vi "DisplayConfig.vi"(9 "EnableSounds":bool) -> (4 "ScoreIP":string, 6 "Cancelled?":bool, 8 "TimerIP":string, 10 "EnableSounds out":bool, 15 "Score Behavior OUT":T1(ring))   [LabVIEW 2013]
uses:
  <vilib>/httpClient/LabVIEWHTTPClient.lvlib
panel:
  in  "Tab Control":enum32{"Page 1", "Page 2"}(tab)
  in  "Tab Control 2":enum32{"Basic Settings", "Advanced"}(tab)
  in  "IP Address (ex:  127.0.0.1)":string="127.0.0.1"
  in  "Check IP Button":bool
  in  "Port (ex:  8008)":string="8008"
  in  "Configure Sound Button":bool
  in  "Score Behavior":T1(ring)
  in  "Timer IP Addr":string="127.0.0.1"
  in  "MultiHomed Timer":bool
  in  "Process Stop Button":bool
  in  "OK Button":bool
  out "Instructions":string="This is the Display Application configuration utility for the FIRST LEGO League Tournament Software.  \n\nPlease type in the IP Address of the server system in the IP Address box to the left and press the \"Check\" button to verify that the server is running.  \"127.0.0.1\" is the default address for launching this application on the SERVER machine itself.  On the SERVER machine, the IP address can be found in the \"Monitor\" page at the bottom left.\n\nOnce you close this page, you can open this back up by pressing the ESC key.  You can press the SPACEBAR to make the display application expand the page, but the page MUST be on a display that is exactly 1024x768.\n\nThe display, by default, will show negative scores as ZERO while maintaining the negative value (for ranking purposes) within the software.  To show negatives scores at their true value, change the Score Behavior to reflect this.  \n\nThe display can play sounds similar to the server application.  This is a major hack, please only use this if you're using the standard sounds and don't need to change settings (unless you REALLY feel like you know what you're doing).  Currently sounds are only configured if enabled on initial launch of the display.  Sounds and config are NOT currently shared between the server and display, but the config information may be shared if hosted on the same computer.  Use with caution."
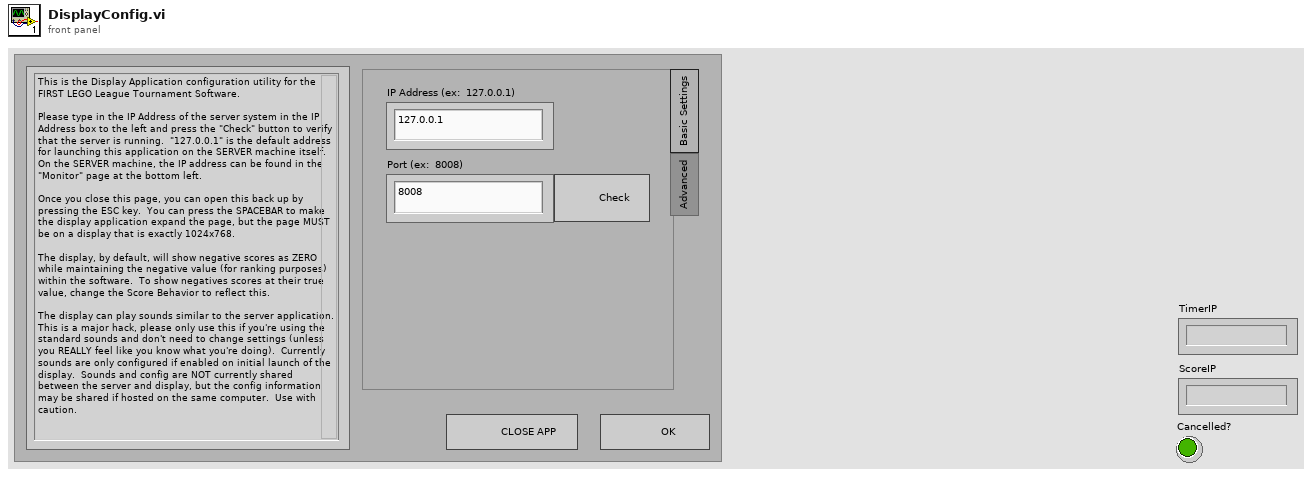
[diagram p1: front panel]
types:
  T1 = enum16{"Show Negative Scores as ZERO", "Show Negative Scores"}
  T2 = enum8{"Enabled", "Disabled", "Disabled and Grayed Out"}
  T3 = typedef "LabVIEWHTTPClient.lvlib/ClientHandle.ctl" = refnum<k1>
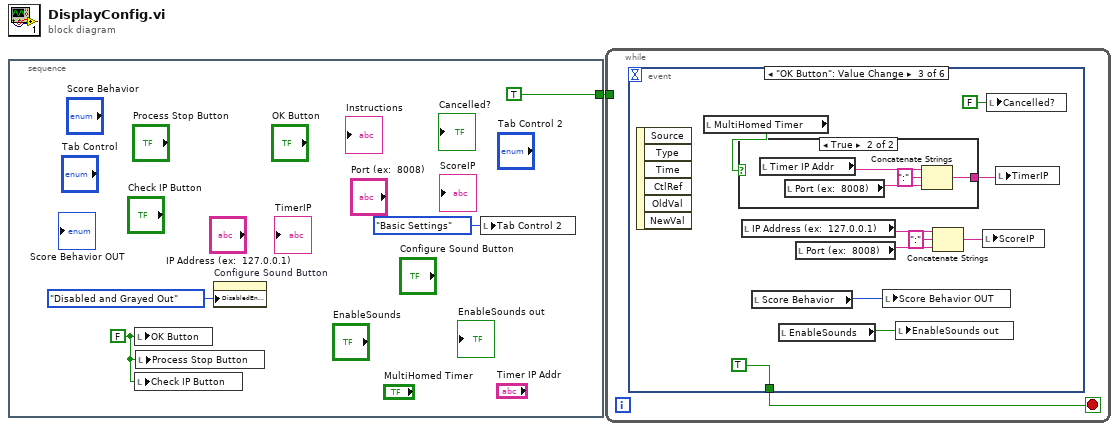
[diagram p0: block diagram]
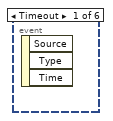
[diagram p2: hidden frame]
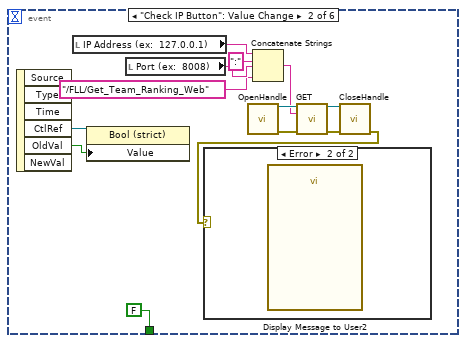
[diagram p3: hidden frame]
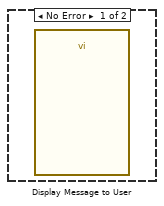
[diagram p4: hidden frame]
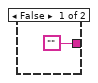
[diagram p5: hidden frame]
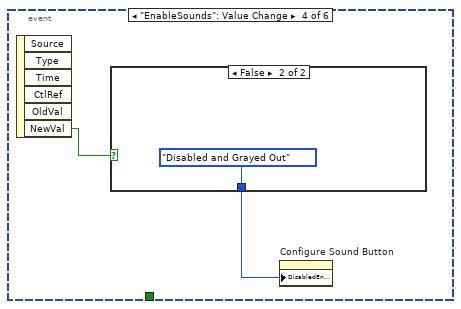
[diagram p6: hidden frame]
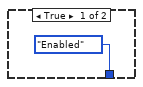
[diagram p7: hidden frame]
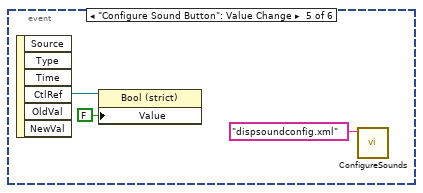
[diagram p8: hidden frame]
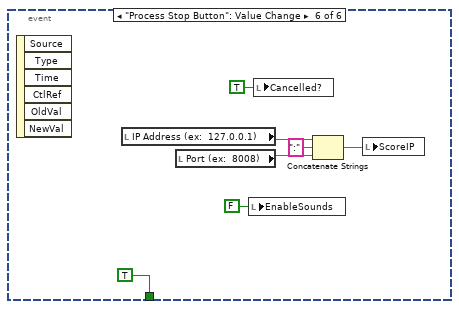
[diagram p9: hidden frame]
diagram:
  n1 = stacked-sequence {
    tunnel: [TRUE] -> w1
    frame #0 {
      w3 = FALSE ("OK Button")
      n2 = local write "OK Button"(w3) -> ()
      n3 = local write "Check IP Button"(w3) -> ()
      n4 = local write "Process Stop Button"(w3) -> ()
      n5 = property on="Configure Sound Button" class="Bool (strict)"("DisabledEnum"=T2."Disabled and Grayed Out" ("Disabled")) -> ()  [unwired: 2 in, 2 out]
      n6 = local write "Tab Control 2"(enum32{"Basic Settings", "Advanced"}."Basic Settings" ("Tab Control 2")) -> ()
    }
  }
  n7 = while {
    tunnel: w1 -> [_]
    stop <- w6 stop-if-true
    n8 = event shown="[2] \"OK Button\": Value Change" {
      selector: _ -> [_ _ _ _ _ _]
      dyn-events: _ -> [_ _ _ _ _ _]
      timeout: _ -> [_ _ _ _ _ _]
      tunnel: [_ FALSE TRUE _ _ TRUE] -> w6
      event Timeout {
        n9 = event-data() -> ()  [unwired: 1 in, 3 out]
      }
      event "Check IP Button": Value Change {
        n10 = event-data() -> ("CtlRef"=w17:refnum<vi>, "OldVal"=w16:bool)  [unwired: 1 in, 4 out]
        n11 = local read "IP Address (ex:  127.0.0.1)"() -> (w15:string)
        n12 = property class="Bool (strict)"(reference=w17, "Value"=w16) -> ()  [unwired: 1 in, 2 out]
        n13 = local read "Port (ex:  8008)"() -> (w13:string)
        n14 = call <vilib>:"OpenHandle.vi"() -> ("client handle out"=w19:T3, "error out"=w18:errorcluster)  [unwired: 14 in]
        n15 = Concatenate Strings(w15, ":" ("string"), w13, "/FLL/Get_Team_Ranking_Web" ("url")) -> (w11:string)
        n16 = call <vilib>:"GET.vi"("client handle"=w19, "url"=w11, "error in (no error)"=w18) -> ("client handle out"=w10:T3, "error out"=w9:errorcluster)  [unwired: 9 in, 2 out]
        n17 = call <vilib>:"CloseHandle.vi"("client handle"=w10, "error in (no error)"=w9) -> ("error out"=w8:errorcluster)  [unwired: 13 in]
        n18 = case shown="Error" w8 {
          frame No Error {
            n19 = call "Display Message to User"() -> ()  [unwired: 10 in, 2 out]
          }
          frame Error {
            n20 = call "Display Message to User2"() -> ()  [unwired: 10 in, 2 out]
          }
        }
      }
      event "OK Button": Value Change {
        n21 = event-data() -> ()  [unwired: 1 in, 6 out]
        n22 = local read "MultiHomed Timer"() -> (w20:bool)
        n23 = case shown="True" w20 {
          tunnel: ["" w34] -> w21
          frame False {
          }
          frame True {
            n24 = local read "Timer IP Addr"() -> (w31:string)
            n25 = local read "Port (ex:  8008)"() -> (w32:string)
            n26 = Concatenate Strings(w31, ":" ("string"), w32) -> (w34:string)
          }
        }
        n27 = local read "IP Address (ex:  127.0.0.1)"() -> (w28:string)
        n28 = local read "Score Behavior"() -> (w23:T1)
        n29 = local read "EnableSounds"() -> (w22:bool)
        n30 = local read "Port (ex:  8008)"() -> (w27:string)
        n31 = local write "Score Behavior OUT"(w23) -> ()
        n32 = local write "EnableSounds out"(w22) -> ()
        n33 = Concatenate Strings(w28, ":" ("string"), w27) -> (w25:string)
        n34 = local write "ScoreIP"(w25) -> ()
        n35 = local write "Cancelled?"(FALSE ("Cancelled?")) -> ()
        n36 = local write "TimerIP"(w21) -> ()
      }
      event "EnableSounds": Value Change {
        n37 = event-data() -> ("NewVal"=w36:bool)  [unwired: 1 in, 5 out]
        n38 = case shown="False" w36 {
          tunnel: [T2."Enabled" ("Disabled") T2."Disabled and Grayed Out" ("Disabled")] -> w35
          frame True {
          }
          frame False {
          }
        }
        n39 = property on="Configure Sound Button" class="Bool (strict)"("DisabledEnum"=w35) -> ()  [unwired: 2 in, 2 out]
      }
      event "Configure Sound Button": Value Change {
        n40 = event-data() -> ("CtlRef"=w40:refnum<vi>)  [unwired: 1 in, 5 out]
        n41 = property class="Bool (strict)"(reference=w40, "Value"=FALSE) -> ()  [unwired: 1 in, 2 out]
        n42 = call "ConfigureSounds.vi"("File"="dispsoundconfig.xml") -> ()  [unwired: 9 in, 2 out]
      }
      event "Process Stop Button": Value Change {
        n43 = event-data() -> ()  [unwired: 1 in, 6 out]
        n44 = local read "IP Address (ex:  127.0.0.1)"() -> (w47:string)
        n45 = local read "Port (ex:  8008)"() -> (w46:string)
        n46 = local write "EnableSounds"(FALSE ("EnableSounds")) -> ()
        n47 = local write "Cancelled?"(TRUE ("Cancelled?")) -> ()
        n48 = Concatenate Strings(w47, ":" ("string"), w46) -> (w44:string)
        n49 = local write "ScoreIP"(w44) -> ()
      }
    }
  }
